vi "LVClass_CorrectionDataManager SetPupilMask.vi"(0 "CorrectionDataManager in":refnum<class "CorrectionDataManager.lvclass">, 5 "Pupil in":refnum<class "Pupil.lvclass">, 11 "error in (no error)":errorcluster) -> (4 "CorrectionDataManager out":refnum<class "CorrectionDataManager.lvclass">, 6 "Pupil out":refnum<class "Pupil.lvclass">, 15 "error out":errorcluster)   [LabVIEW 2020, in "CorrectionDataManager.lvclass"]
doc: "Command matrix computation preferences.\n\n--------------------------------------------------------------------------------\n\n<B>corrdata_managerIn </B> : CorrDataManager object.\n<B>corrdata_managerOut </B> : CorrDataManager object.\n<B>nb_kept_modes </B> : Number of influences (starting from the highest) to keep.\n<B>tilt_filtering </B> : If True, computed command matrix does not take tilt into account.\n<B>ErrorIn </B> : Error\n<B>ErrorOut </B> : Error\n\n--------------------------------------------------------------------------------"
uses:
  CorrectionDataManager.lvclass
  Pupil.lvclass
  LVClass_Pupil Read Pupil.vi
  LVClass_CorrectionDataManager Read CorrectionDataManager.vi
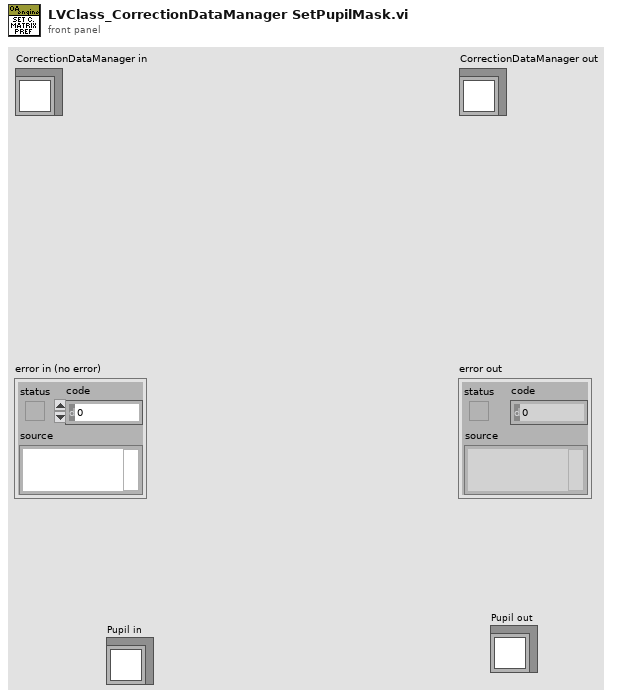
[diagram p1: front panel]
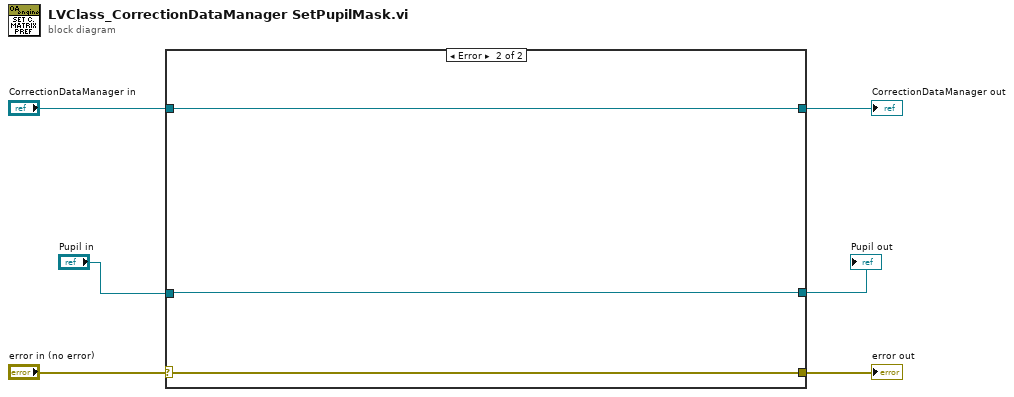
[diagram p0: block diagram]
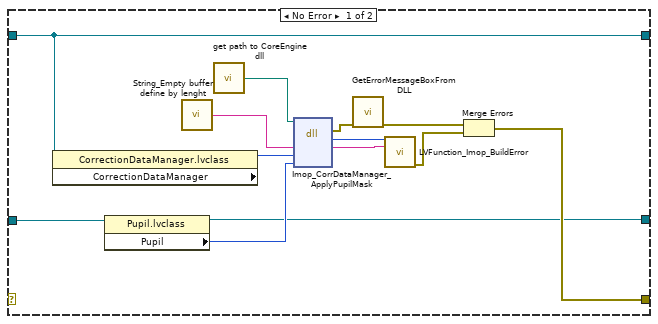
[diagram p2: hidden frame]
diagram:
  n1 = case shown="Error" "error in (no error)" {
    selector: "error in (no error)" -> [_ w22]
    tunnel: [w11 w22] -> w5
    tunnel: [w12 w21] -> w6
    tunnel: "CorrectionDataManager in" -> [w12 w21]
    tunnel: "Pupil in" -> [w9 w20]
    tunnel: [w7 w20] -> w1
    frame No Error {
      n2 = property class="CorrectionDataManager.lvclass"(reference=w12) -> ("CorrectionDataManager"=w10:i32)  [unwired: 1 in, 2 out]
      n3 = property class="Pupil.lvclass"(reference=w9) -> (reference out=w7:refnum<class "Pupil.lvclass">, "Pupil"=w8:i32)  [unwired: 1 in, 1 out]
      n4 = call "String_Empty buffer define by lenght.vi"() -> ("Empty buffer"=w17:string)  [unwired: 1 in]
      n5 = call "get path to CoreEngine dll.vi"() -> ("path to c_interface_vc100.dll"=w16:path)  [unwired: 12 in, 3 out]
      n6 = dll-call lib="D:/soft/HASO_v3/SVN_trunk/ImOpCoreEngine4_LV2011/DLLs/c_interface_vc100.dll" fn="Imop_CorrDataManager_ApplyPupilMask"(path in=w16, "message"=w17, "WavefrontCorrection"=w10, "pupil"=w8) -> (error out=w15:errorcluster, "return type"=w19:i32, "message"=w18:string)  [unwired: 4 in, 1 out]
      n7 = call "GetErrorMessageBoxFromDLL.vi"("error IN"=w15) -> ("error OUT"=w14:errorcluster)  [unwired: 10 in]
      n8 = call "LVFunction_Imop_BuildError.vi"("code"=w19, "String to Prepend to source (\"\")"=w18) -> ("error out"=w13:errorcluster)  [unwired: 13 in]
      n9 = Merge Errors(w14, w13) -> (w11:errorcluster)
    }
    frame Error {
    }
  }
  "error out" <- w5
  "CorrectionDataManager out" <- w6
  "Pupil out" <- w1
